vi "01_integration_time.vi"() -> ()   [LabVIEW 2022 SP3]
panel:
  in  "stop":bool
  in  "Integration Time (us)":dbl=10000.0
  out "Number of Spectrometers":i32
  out "?":T1(graph)
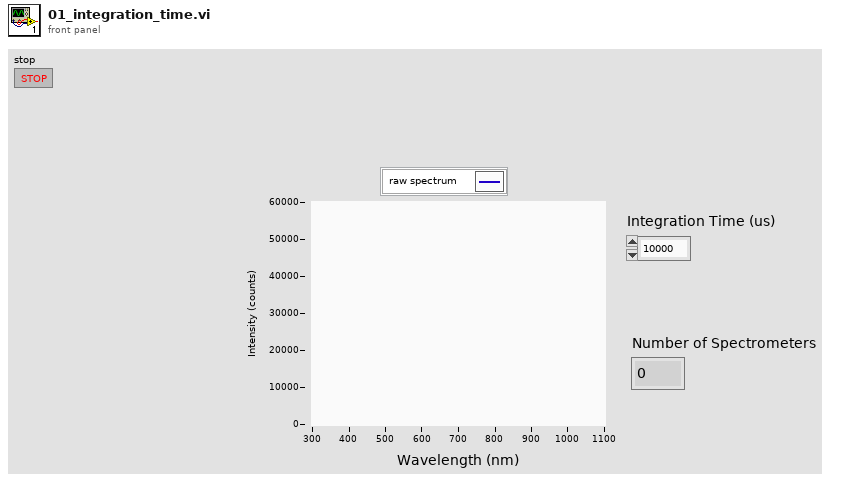
[diagram p1: front panel]
types:
  T1 = cluster{"WL Values":dbl[], "Spectrum Values":dbl[]}
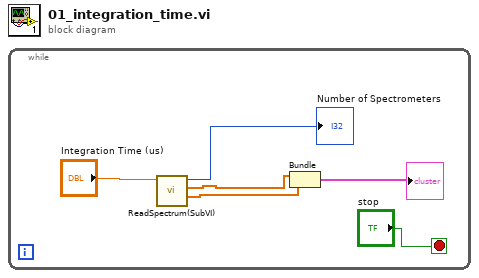
[diagram p0: block diagram]
diagram:
  n1 = while {
    stop <- "stop" stop-if-true
    n2 = call "ReadSpectrum(SubVI).vi"("Enter the \nInetegration Time"="Integration Time (us)") -> ("Spectrum Values"=w6:dbl[], "WL Values"=w5:dbl[], "Number of Spectrometers"=→"Number of Spectrometers":i32)  [unwired: 8 in]
    n3 = Bundle("WL Values"=w5, "Spectrum Values"=w6) -> (→"?":T1)  [unwired: 1 in]
  }
